vi "cali_write cali array.vi"(6 "ROI cali array":dbl[][](array[numeric]), 7 "beads info in":T1[](array[typedef]), 10 "校准步数":refnum<vi>, 11 "校准第几步":refnum<vi>) -> (2 "beads info out":T1[](array[typedef]))   [LabVIEW 2017]
uses:
  control/bead info.ctl
  <vilib>/vision/Image Controls.llb/IMAQ Image.ctl
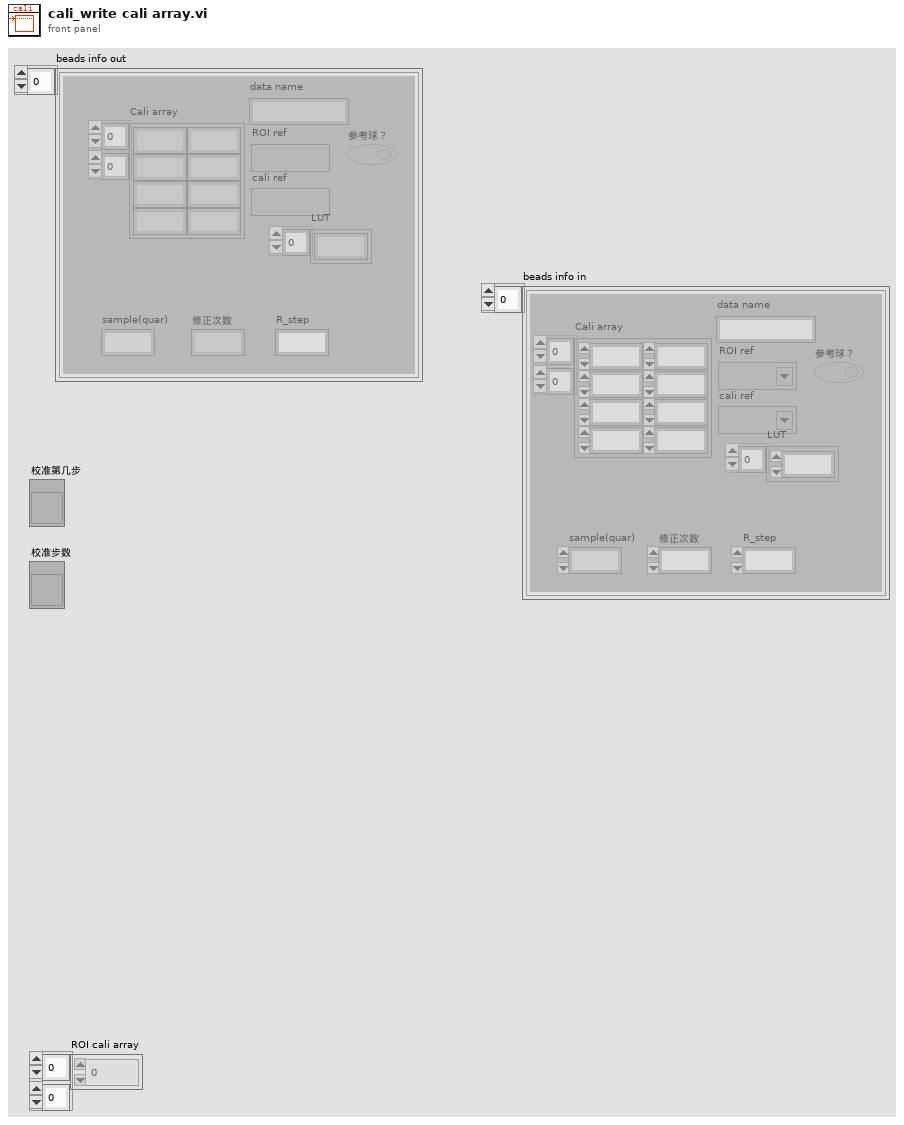
[diagram p1: front panel]
types:
  T1 = typedef "bead info.ctl" = cluster{"data name":string, "ROI ref":T2, "cali ref":T2, "参考球？":bool, "LUT":dbl[], "Cali array":dbl[][], "修正次数":i32, "R_step":dbl, "sample(quar)":i32}
  T2 = typedef "IMAQ Image.ctl" = refnum<image>
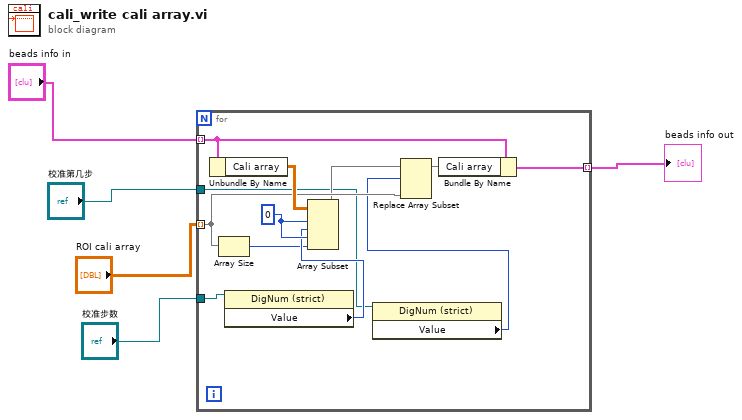
[diagram p0: block diagram]
diagram:
  n1 = for "For循环" {
    tunnel: "ROI cali array" -> [w12] mode=indexing
    tunnel: "beads info in" -> [w17] mode=indexing
    tunnel: [w15] -> w2 mode=indexing
    tunnel: "校准第几步" -> [w7]
    tunnel: "校准步数" -> [w6]
    w13 = 0 ("索引")
    n2 = Unbundle By Name(w17) -> ("Cali array"=w14:dbl[][])
    n3 = Array Size(array=w12) -> (size(s)=w9:i32)
    n4 = property class="DigNum (strict)"(reference=w6) -> ("Value"=w10:i32)  [unwired: 1 in, 2 out]
    n5 = Array Subset(array=w14, index (row)=w13, length (row)=w10, index (col)=w13, length (col)=w9) -> (w11:dbl[][])
    n6 = property class="DigNum (strict)"(reference=w7) -> ("Value"=w8:i32)  [unwired: 1 in, 2 out]
    n7 = Replace Array Subset(array=w11, new element=w12, index (row)=w8) -> (w16:dbl[][])  [unwired: 1 in]
    n8 = Bundle By Name(cluster=w17, "Cali array"=w16) -> (w15:T1)
  }
  "beads info out" <- w2
